vi "ConvertGoop3ToGoop4_SelectNodesToBeInsideIP.vi"(1 "NodesIn":cluster{"NodesIn":T3[]}[](array[cluster]), 5 "BundleNodes":cluster{"BundleNodes":refnum<vi>[]}[](array[cluster]), 9 "BundleNodeTypes":cluster{"BundleNodeTypes":string[]}[](array[cluster]), 11 "error in":errorcluster, 12 "GetAttribute_AttributeTerminal":refnum<vi>[](array[refnum]), 13 "FirstGetAttributesDrainsTerminals":refnum<vi>[](array[refnum]), 14 "LastGetAttributesSourceTerminals":refnum<vi>[](array[refnum])) -> (4 "NodesOut":cluster{"NodesIn":T3[]}[](array[cluster]), 6 "IPE-Position":T1, 8 "IPE-Frame Size":T2, 15 "error out":errorcluster)   [LabVIEW 2014]
uses:
  <resource>/Framework/Providers/Open_GDS/ClassProviders/Common/ScriptingFunctions/Scripting_NodeInfo.ctl
  <vilib>/Utility/miscctls.llb/LVBoundsTypeDef.ctl
  <vilib>/Utility/miscctls.llb/LVPositionTypeDef.ctl
panel:
  in  "SetAttributesDrainsTerminals":refnum<vi>[](array[refnum])
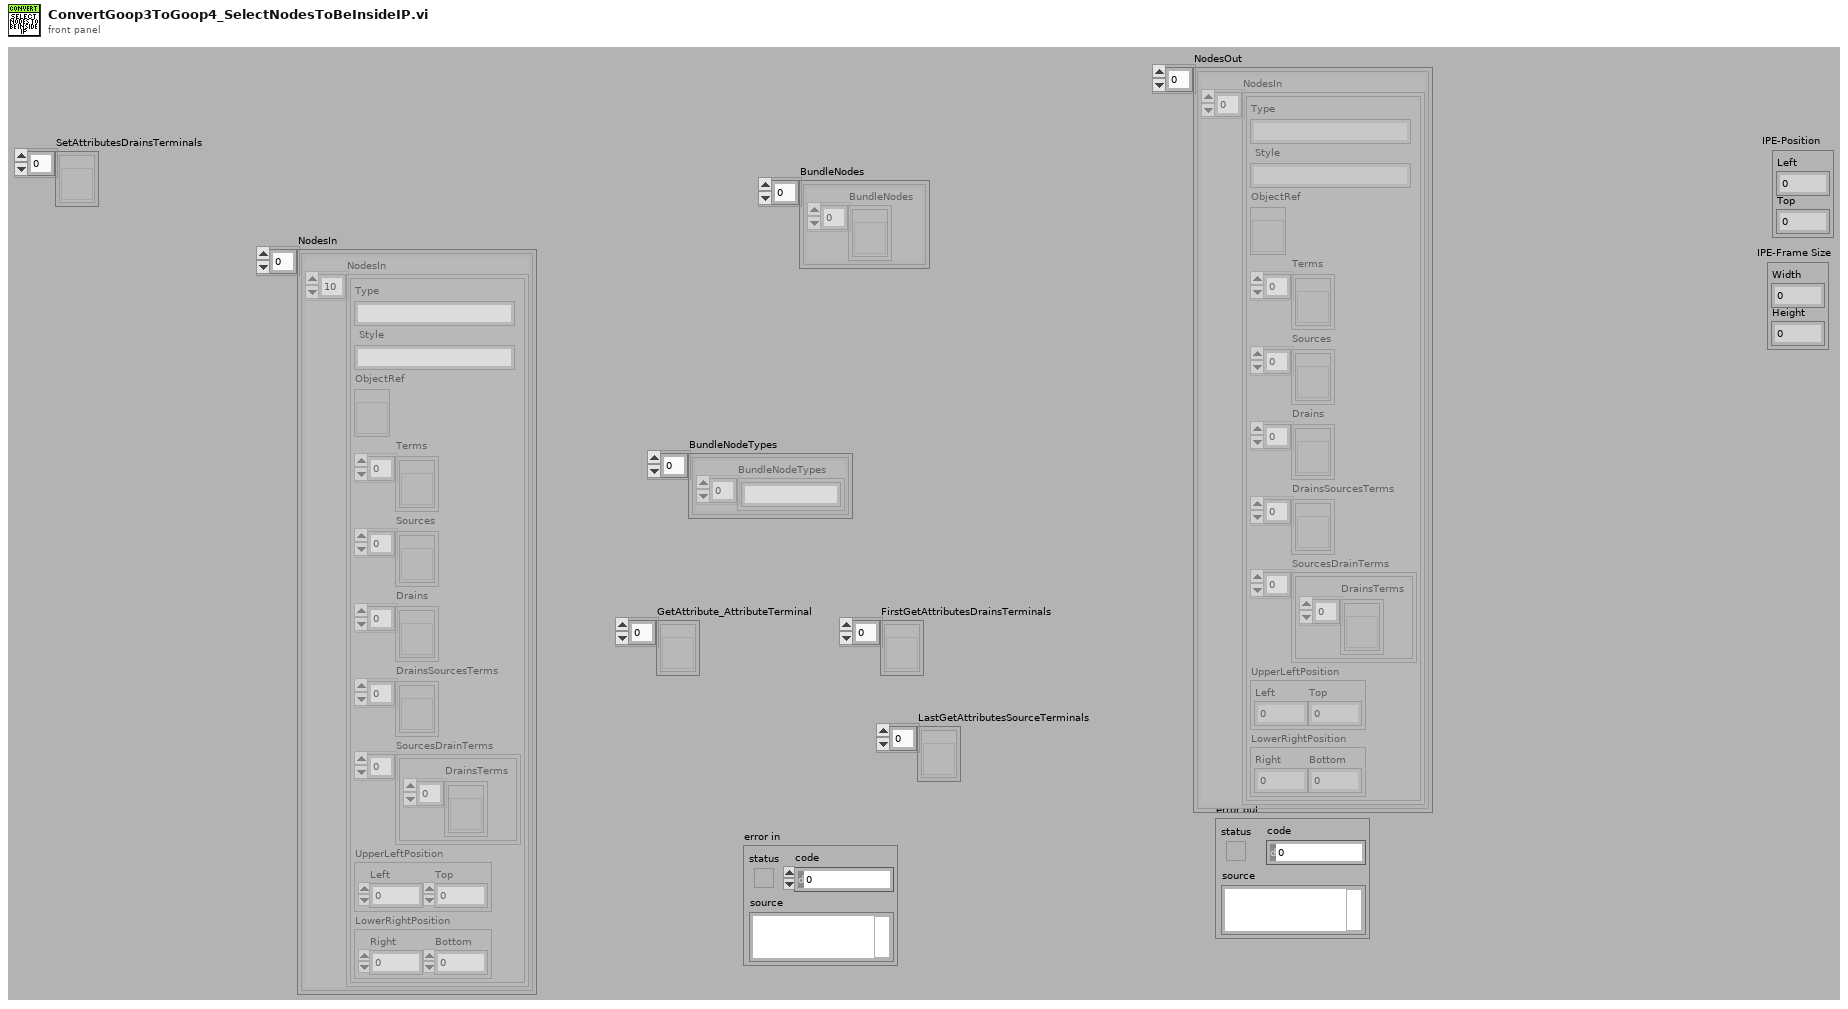
[diagram p1: front panel]
types:
  T1 = typedef "LVPositionTypeDef.ctl" = cluster{"Left":i32, "Top":i32}
  T2 = typedef "LVBoundsTypeDef.ctl" = cluster{"Width":u32, "Height":u32}
  T3 = typedef "Scripting_NodeInfo.ctl" = cluster{"Type":string, "Style":string, "ObjectRef":refnum<vi>, "Terms":refnum<vi>[], "Sources":refnum<vi>[], "Drains":refnum<vi>[], "DrainsSourcesTerms":refnum<vi>[], "SourcesDrainTerms":cluster{"DrainsTerms":refnum<vi>[]}[], "UpperLeftPosition":cluster{"Left":i32, "Top":i32}, "LowerRightPosition":cluster{"Right":i32, "Bottom":i32}}
  T4 = cluster{"SourcesDrainTerms":cluster{"DrainsTerms":refnum<vi>[]}[]}[]
  T5 = cluster{"SourcesDrainTerms":cluster{"DrainsTerms":refnum<vi>[]}[]}
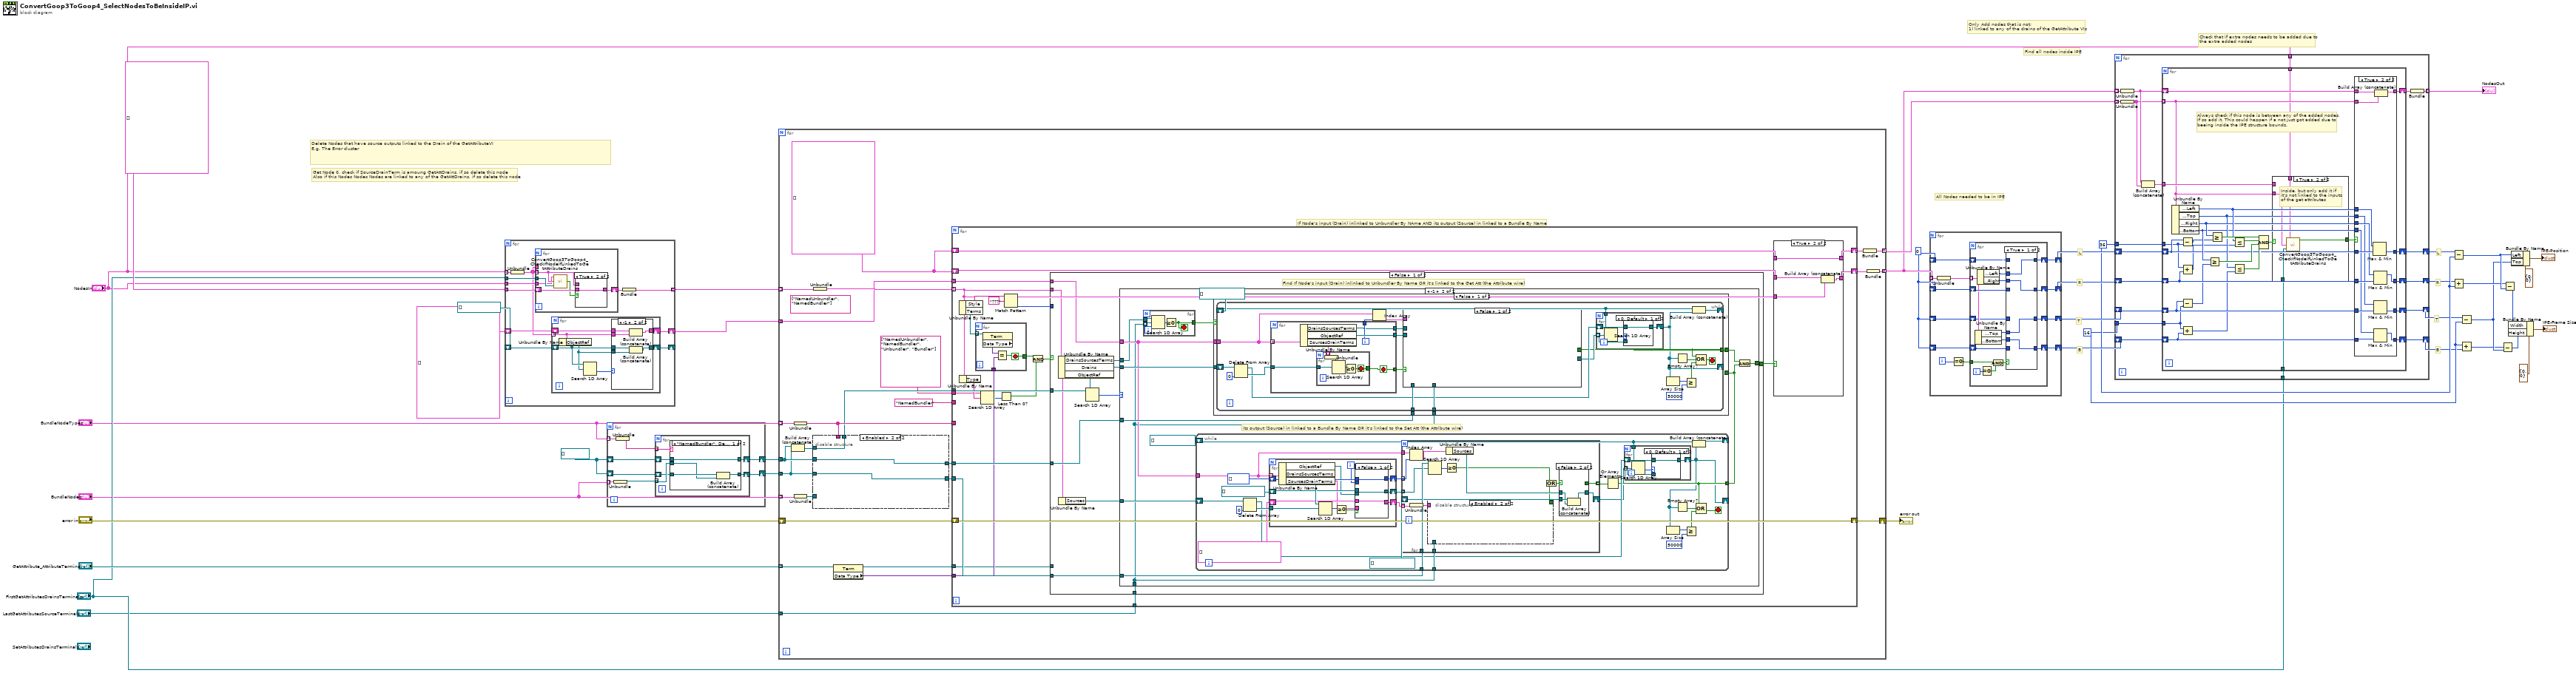
[diagram p0: block diagram]
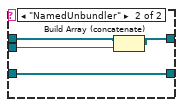
[diagram p2: hidden frame]
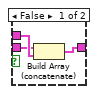
[diagram p4: hidden frame]
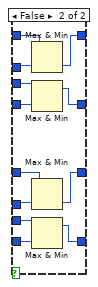
[diagram p7: hidden frame]
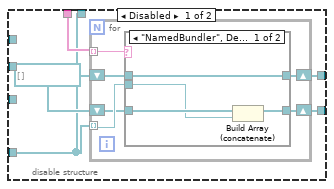
[diagram p8: hidden frame]
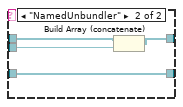
[diagram p9: hidden frame]
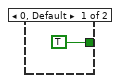
[diagram p10: hidden frame]
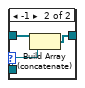
[diagram p11: hidden frame]
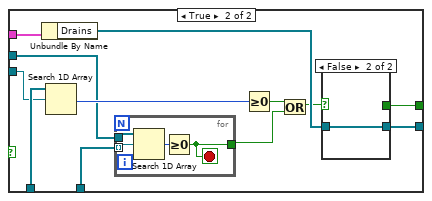
[diagram p12: hidden frame]
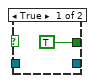
[diagram p13: hidden frame]
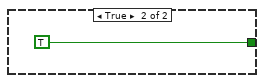
[diagram p14: hidden frame]
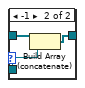
[diagram p15: hidden frame]
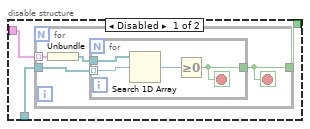
[diagram p16: hidden frame]
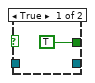
[diagram p17: hidden frame]
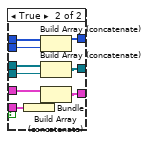
[diagram p18: hidden frame]
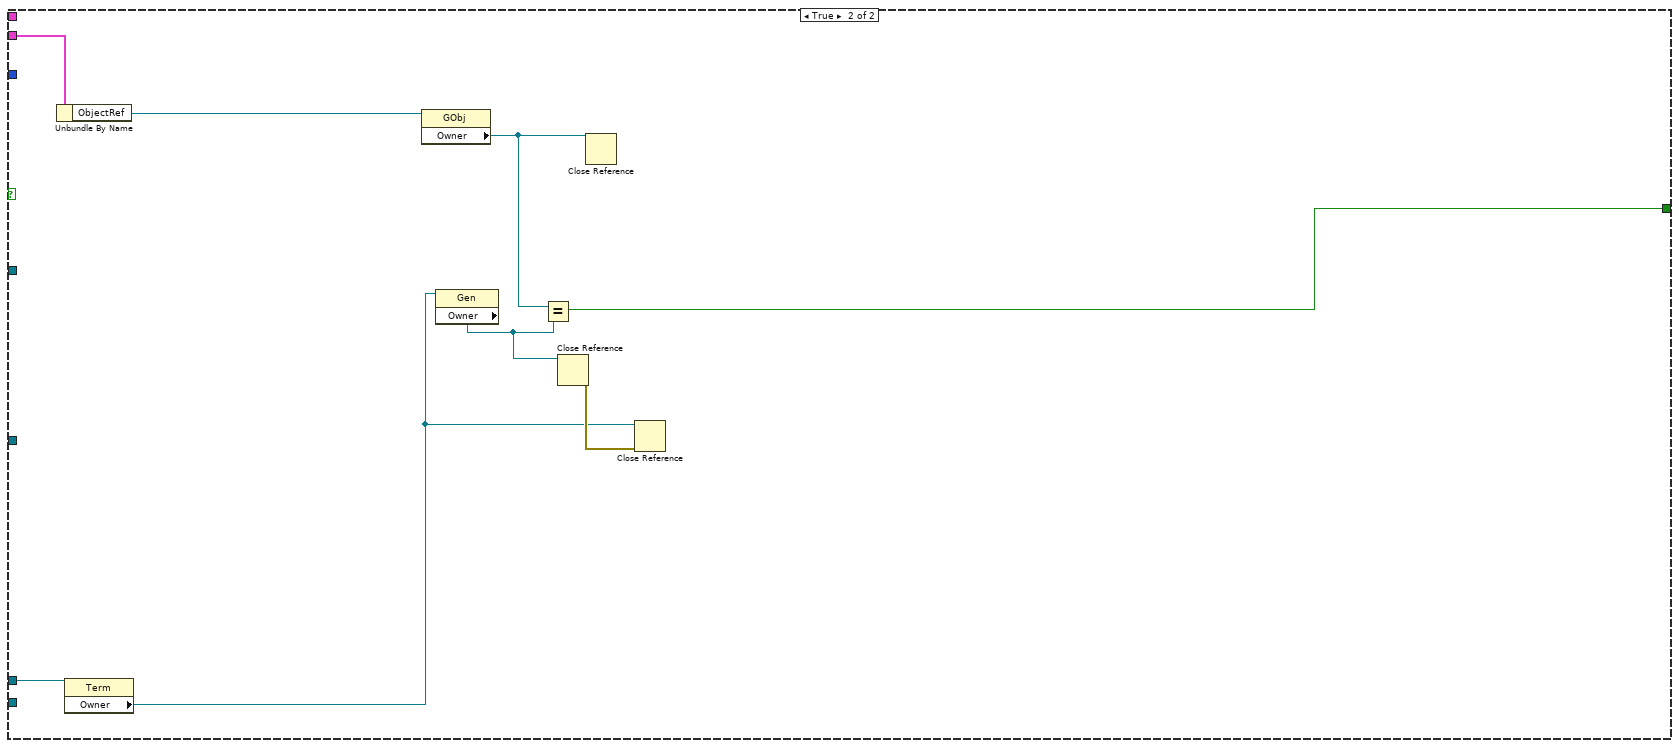
[diagram p19: hidden frame]
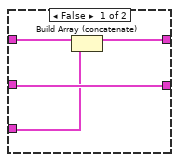
[diagram p20: hidden frame]
diagram:
  w7 = refnum<vi>[] []
  w19 = 16 ("y")
  w26 = 36 ("y")
  w15 = 0 ("Right")
  # "Get Node 0, check if SourceDrainTerm is amoung GetAttDrains, if so delete this node\nAlso if this Nodes Nodes Nodes are linked to any of the GetAttDrains, if so delete this node"
  # "Delete Nodes that have source outputs linked to the Drain of the GetAttributeVI\nE.g. The Error cluster"
  # "Check that if extra nodes needs to be added due to\nthe extra added nodes"
  # "Only Add nodes that is not:\n1) linked to any of the drains of the GetAttribute VIs"
  # "B"
  # "T"
  # "R"
  # "L"
  # "Find all nodes inside IPE"
  # "B"
  # "T"
  # "R"
  # "L"
  # "All Nodes needed to be in IPE"
  n1 = for {
    tunnel: "NodesIn" -> [w51] mode=indexing
    tunnel: [w49] -> w13 mode=indexing
    tunnel: T3[] [] -> [w48]
    tunnel: "FirstGetAttributesDrainsTerminals" -> [w47]
    tunnel: "NodesIn" -> [w46]
    shift-right: [w45] -> w2
    shift-left: T3[] [] -> [w44]
    shift-right: [w42] -> _
    shift-left: refnum<vi>[] [] -> [w43]
    n2 = Unbundle(w51) -> ("NodesIn"=w41:T3[])
    n3 = for {
      tunnel: w41 -> [w72] mode=indexing
      shift-right: [w71] -> w50
      shift-left: w48 -> [w70]
      tunnel: w41 -> [_]
      tunnel: w47 -> [w68]
      tunnel: w46 -> [w67]
      n4 = call <resource>:"ConvertGoop3ToGoop4_CheckIfNodeIfLinkedToGetAttributeDrains.vi"("FirstGetAttributesDrainsTerminals"=w68, "NodeInfo"=w72, "NodesIn"=w67) -> ("Boolean"=w69:bool)
      n5 = case shown="True" w69 {
        tunnel: w72 -> [w75 _]
        tunnel: [w74 w76] -> w71
        tunnel: w70 -> [w73 w76]
        frame False {
          n6 = Build Array (concatenate)(w73, w75) -> (w74:T3[])
        }
        frame True {
        }
      }
    }
    n7 = for {
      tunnel: w41 -> [w55] mode=indexing
      shift-right: [w58] -> w45
      shift-left: w44 -> [w57]
      shift-right: [w56] -> w42
      shift-left: w43 -> [w54]
      n8 = Unbundle By Name(w55) -> ("ObjectRef"=w53:refnum<vi>)
      n9 = Search 1D Array(1D array=w54, element=w53) -> (index of element=w52:i32)  [unwired: 1 in]
      n10 = case shown="-1" w52 {
        tunnel: [w60 w66] -> w58
        tunnel: w57 -> [w60 w65]
        tunnel: [w59 w64] -> w56
        tunnel: w55 -> [_ w63]
        tunnel: w54 -> [w59 w62]
        tunnel: w53 -> [_ w61]
        frame 0, Default {
        }
        frame -1 {
          n11 = Build Array (concatenate)(w65, w63) -> (w66:T3[])
          n12 = Build Array (concatenate)(w62, w61) -> (w64:refnum<vi>[])
        }
      }
    }
    n13 = Bundle(w50) -> (w49:cluster{T3[]})  [unwired: 1 in]
  }
  n14 = for {
    tunnel: "BundleNodes" -> [w84] mode=indexing
    shift-right: [w80] -> w5
    shift-left: w7 -> [w82]
    shift-right: [w79] -> w4
    shift-left: w7 -> [w81]
    tunnel: "BundleNodeTypes" -> [w78] mode=indexing
    n15 = Unbundle(w84) -> ("BundleNodes"=w83:refnum<vi>[])
    n16 = Unbundle(w78) -> ("BundleNodeTypes"=w77:string[])
    n17 = for {
      tunnel: w77 -> [w90] mode=indexing
      tunnel: w83 -> [w87] mode=indexing
      shift-right: [w88] -> w80
      shift-left: w82 -> [w89]
      shift-right: [w86] -> w79
      shift-left: w81 -> [w85]
      n18 = case shown="\"NamedBundler\", Default" w90 {
        tunnel: w89 -> [w94 w98]
        tunnel: [w94 w97] -> w88
        tunnel: w87 -> [w91 w96]
        tunnel: w85 -> [w93 w95]
        tunnel: [w92 w95] -> w86
        frame "NamedBundler", Default {
          n19 = Build Array (concatenate)(w93, w91) -> (w92:refnum<vi>[])
        }
        frame "NamedUnbundler" {
          n20 = Build Array (concatenate)(w98, w96) -> (w97:refnum<vi>[])
        }
      }
    }
  }
  n21 = for {
    tunnel: w13 -> [w119] mode=indexing
    tunnel: "BundleNodeTypes" -> [w117] mode=indexing
    tunnel: "BundleNodes" -> [w115] mode=indexing
    tunnel: [w110] -> w39 mode=indexing
    tunnel: [w112] -> w36 mode=indexing
    shift-right: [w124] -> w40
    shift-left: "error in" -> [w120]
    tunnel: "GetAttribute_AttributeTerminal" -> [w109] mode=indexing
    tunnel: "LastGetAttributesSourceTerminals" -> [w106]
    tunnel: w5 -> [w105]
    tunnel: w4 -> [w104]
    tunnel: w2 -> [w101]
    (unwired) string[] ["NamedUnbundler", "NamedBundler"]
    w121 = T3[] []
    # "If Node's input (Drain) inlinked to Unbundler By NAme AND its output (Source) in linked to a Bundle By Name"
    n22 = Build Array (concatenate)(w105, w104) -> (w103:refnum<vi>[])
    n23 = Unbundle(w117) -> ("BundleNodeTypes"=w116:string[])
    n24 = Unbundle(w115) -> ("BundleNodes"=w114:refnum<vi>[])
    n25 = disable-structure shown="Enabled" {
      disable-tunnel: [w128 w146] -> w123
      disable-tunnel: [w127 w145] -> w122
      disable-tunnel: w116 -> [w126 _]
      disable-tunnel: w114 -> [w125 _]
      disable-tunnel: w105 -> [_ w146]
      disable-tunnel: w104 -> [_ w145]
      disable-tunnel: w103 -> [_ w144]
      disable-tunnel: [w125 w144] -> w102
      frame Disabled {
        w129 = refnum<vi>[] []
        n26 = for {
          tunnel: w126 -> [w135] mode=indexing
          tunnel: w125 -> [w132] mode=indexing
          shift-right: [w133] -> w128
          shift-left: w129 -> [w134]
          shift-right: [w131] -> w127
          shift-left: w129 -> [w130]
          n27 = case shown="\"NamedBundler\", Default" w135 {
            tunnel: w134 -> [w139 w143]
            tunnel: [w139 w142] -> w133
            tunnel: w132 -> [w136 w141]
            tunnel: w130 -> [w138 w140]
            tunnel: [w137 w140] -> w131
            frame "NamedBundler", Default {
              n28 = Build Array (concatenate)(w138, w136) -> (w137:refnum<vi>[])
            }
            frame "NamedUnbundler" {
              n29 = Build Array (concatenate)(w143, w141) -> (w142:refnum<vi>[])
            }
          }
        }
      }
      frame Enabled {
      }
    }
    n30 = Unbundle(w119) -> (w118:T3[])
    n31 = property class="Term"(reference=w109) -> (reference out=w107:refnum<vi>, "Data Type"=w108:variant)  [unwired: 1 in, 1 out]
    n32 = for {
      tunnel: w118 -> [w153] mode=indexing
      tunnel: w116 -> [_]
      shift-right: [w170] -> w124
      shift-left: w120 -> [w170]
      shift-right: [w169] -> w113
      shift-left: w121 -> [w168]
      tunnel: w101 -> [w167]
      tunnel: w123 -> [w166]
      tunnel: w122 -> [w163]
      tunnel: w102 -> [w164]
      shift-right: [w162] -> w111
      shift-left: w121 -> [w161]
      tunnel: w108 -> [w159]
      tunnel: w107 -> [w158]
      tunnel: w106 -> [w157]
      tunnel: "NamedBundler" ("regular expression") -> [_]
      tunnel: string[] ["NamedUnbundler", "NamedBundler", "Unbundler", "Bundler"] -> [w149]
      n33 = Unbundle By Name(w153) -> ("Style"=w156:string, "Terms"=w160:refnum<vi>[])
      n34 = Unbundle By Name(w153) -> ("Type"=w150:string)
      n35 = for {
        tunnel: w160 -> [w371] mode=indexing
        tunnel: w159 -> [w369]
        tunnel: [w368] -> w152
        stop <- w368 stop-if-true
        n36 = property class="Term"(reference=w371) -> ("Data Type"=w370:variant)  [unwired: 1 in, 2 out]
        n37 = Equal?(x=w370, y=w369) -> (x = y?=w368:bool)
      }
      n38 = Search 1D Array(1D array=w149, element=w150) -> (index of element=w148:i32)  [unwired: 1 in]
      n39 = Less Than 0?(x=w148) -> (x < 0?=w147:bool)
      n40 = Match Pattern(string=w156, regular expression="???") -> (offset past match=w154:i32)  [unwired: 1 in, 3 out]
      n41 = And(x=w152, y=w147) -> (x .and. y?=w151:bool)
      n42 = case shown="False" w151 {
        tunnel: w167 -> [w181 _]
        tunnel: w166 -> [w180 _]
        tunnel: [w179 w364] -> w165
        tunnel: w164 -> [w178 _]
        tunnel: w163 -> [w174 _]
        tunnel: w153 -> [w173 w367]
        tunnel: w158 -> [_ w365]
        tunnel: w157 -> [w171 _]
        tunnel: w154 -> [_ _]
        frame False {
          # "Find If Node's input (Drain) inlinked to Unbundler By Name OR it's linked to the Get Att (the Attribute wire)"
          n43 = Unbundle By Name(w173) -> ("DrainsSourcesTerms"=w172:refnum<vi>[], "Drains"=w182:refnum<vi>[], "ObjectRef"=w177:refnum<vi>)
          n44 = Unbundle By Name(w173) -> ("Sources"=w175:refnum<vi>[])
          n45 = Search 1D Array(1D array=w178, element=w177) -> (index of element=w176:i32)  [unwired: 1 in]
          n46 = case shown="-1" w176 {
            tunnel: w182 -> [_ w195]
            tunnel: w181 -> [_ w192]
            tunnel: w180 -> [_ w193]
            tunnel: [TRUE w194] -> w179
            tunnel: w175 -> [_ w191]
            tunnel: w174 -> [_ w190]
            tunnel: w172 -> [_ w188]
            tunnel: w171 -> [_ w186]
            frame 0, Default {
            }
            frame -1 {
              # "its output (Source) in linked to a Bundle By Name OR it's linked to the Set Att (the Attribute wire)"
              n47 = for {
                tunnel: w188 -> [w267]
                tunnel: w186 -> [w266] mode=indexing
                tunnel: [w264] -> w187
                stop <- w264 stop-if-true
                n48 = Search 1D Array(1D array=w267, element=w266) -> (index of element=w265:i32)  [unwired: 1 in]
                n49 = Greater Or Equal To 0?(x=w265) -> (x >= 0?=w264:bool)
              }
              n50 = while {
                tunnel: w192 -> [w287]
                tunnel: w190 -> [w292]
                tunnel: [w270] -> w185
                shift-right: [w269] -> _
                shift-left: w191 -> [w291]
                tunnel: w186 -> [w279]
                shift-right: [w278] -> _
                shift-left: refnum<vi>[] [] -> [w277]
                stop <- w271 stop-if-true
                n51 = Delete From Array(array=w291, index=0) -> (deleted portion=w288:refnum<vi>, array with subset deleted=w276:refnum<vi>[])  [unwired: 1 in]
                n52 = for {
                  tunnel: w287 -> [w346] mode=indexing
                  tunnel: w288 -> [w345]
                  shift-right: [w341] -> w286
                  shift-left: i32[] [] -> [w340]
                  shift-right: [w338] -> w285
                  shift-left: refnum<vi>[] [] -> [w339]
                  shift-right: [w333] -> w280
                  shift-left: T4 [] -> [w335]
                  i -> [w337]
                  n53 = Unbundle By Name(w346) -> ("ObjectRef"=w336:refnum<vi>, "DrainsSourcesTerms"=w343:refnum<vi>[], "SourcesDrainTerms"=w334:cluster{"DrainsTerms":refnum<vi>[]}[])
                  n54 = Search 1D Array(1D array=w343, element=w345) -> (index of element=w344:i32)  [unwired: 1 in]
                  n55 = Greater Or Equal To 0?(x=w344) -> (x >= 0?=w342:bool)
                  n56 = case shown="False" w342 {
                    tunnel: [w349 w359] -> w341
                    tunnel: w340 -> [w349 w358]
                    tunnel: w339 -> [w348 w357]
                    tunnel: [w348 w356] -> w338
                    tunnel: w337 -> [_ w355]
                    tunnel: w336 -> [_ w354]
                    tunnel: w335 -> [w347 w352]
                    tunnel: [w347 w353] -> w333
                    tunnel: w334 -> [_ w351]
                    frame False {
                    }
                    frame True {
                      n57 = Bundle("SourcesDrainTerms"=w351) -> (w350:T5)  [unwired: 1 in]
                      n58 = Build Array (concatenate)(w358, w355) -> (w359:i32[])
                      n59 = Build Array (concatenate)(w357, w354) -> (w356:refnum<vi>[])
                      n60 = Build Array (concatenate)(w352, w350) -> (w353:T4)
                    }
                  }
                }
                n61 = for {
                  tunnel: w292 -> [w317]
                  tunnel: [w316] -> w289 mode=indexing
                  tunnel: w287 -> [w313]
                  tunnel: w286 -> [w312] mode=indexing
                  tunnel: w285 -> [w310] mode=indexing
                  shift-right: [w315] -> w268
                  shift-left: refnum<vi>[] [] -> [w309]
                  tunnel: w280 -> [w305] mode=indexing
                  tunnel: w279 -> [w303]
                  n62 = Unbundle(w305) -> ("SourcesDrainTerms"=w304:cluster{"DrainsTerms":refnum<vi>[]}[])
                  n63 = Index Array(array=w313, index=w312) -> (element=w311:T3)
                  n64 = disable-structure shown="Enabled" {
                    disable-tunnel: w304 -> [w320 _]
                    disable-tunnel: w303 -> [w319 _]
                    disable-tunnel: [w318 _] -> w302
                    frame Disabled {
                      n65 = for {
                        tunnel: w320 -> [w324] mode=indexing
                        tunnel: w319 -> [w322]
                        tunnel: [w321] -> w318
                        stop <- w321 stop-if-true
                        n66 = Unbundle(w324) -> ("DrainsTerms"=w323:refnum<vi>[])
                        n67 = for {
                          tunnel: w323 -> [w328]
                          tunnel: w322 -> [w327] mode=indexing
                          tunnel: [w325] -> w321
                          stop <- w325 stop-if-true
                          n68 = Search 1D Array(1D array=w328, element=w327) -> (index of element=w326:i32)  [unwired: 1 in]
                          n69 = Greater Or Equal To 0?(x=w326) -> (x >= 0?=w325:bool)
                        }
                      }
                    }
                    frame Enabled {
                    }
                  }
                  n70 = Search 1D Array(1D array=w317, element=w310) -> (index of element=w308:i32)  [unwired: 1 in]
                  n71 = Greater Or Equal To 0?(x=w308) -> (x >= 0?=w307:bool)
                  n72 = Unbundle By Name(w311) -> ("Sources"=w314:refnum<vi>[])
                  n73 = Or(x=w307, y=w302) -> (x .or. y?=w306:bool)
                  n74 = case shown="False" w306 {
                    tunnel: [TRUE _] -> w316
                    tunnel: [_ w330] -> w315
                    tunnel: w314 -> [_ w331]
                    tunnel: w309 -> [_ w332]
                    frame True {
                    }
                    frame False {
                      n75 = Build Array (concatenate)(w332, w331) -> (w330:refnum<vi>[])
                    }
                  }
                }
                n76 = Or Array Elements(Boolean array=w289) -> (logical OR=w270:bool)
                n77 = for {
                  shift-right: [w296] -> w269
                  shift-left: w276 -> [w297]
                  tunnel: w268 -> [w295] mode=indexing
                  tunnel: w277 -> [w293]
                  n78 = Search 1D Array(1D array=w293, element=w295) -> (index of element=w294:i32)  [unwired: 1 in]
                  n79 = case shown="0, Default" w294 {
                    tunnel: w297 -> [w298 w301]
                    tunnel: [w298 w300] -> w296
                    tunnel: w295 -> [_ w299]
                    frame 0, Default {
                    }
                    frame -1 {
                      n80 = Build Array (concatenate)(w301, w299) -> (w300:refnum<vi>[])
                    }
                  }
                }
                n81 = Array Size(array=w269) -> (size(s)=w272:i32)
                n82 = Empty Array?(array=w269) -> (empty?=w275:bool)
                n83 = Greater Or Equal?(x=w272, y=50000) -> (x >= y?=w274:bool)
                n84 = Build Array (concatenate)(w277, w269) -> (w278:refnum<vi>[])
                n85 = Compound Arithmetic op=OR(w270, w275, w274) -> (w271:bool)
              }
              n86 = case shown="False" w187 {
                tunnel: w195 -> [w201 _]
                tunnel: w193 -> [w200 _]
                tunnel: w192 -> [w199 _]
                tunnel: [w198 TRUE] -> w189
                tunnel: w186 -> [w197 _]
                tunnel: w185 -> [_ _]
                frame False {
                  n87 = while {
                    tunnel: w199 -> [w217]
                    tunnel: w200 -> [w221]
                    tunnel: [w204] -> w198
                    shift-right: [w202] -> _
                    shift-left: w201 -> [w220]
                    tunnel: w197 -> [w214]
                    shift-right: [w212] -> _
                    shift-left: refnum<vi>[] [] -> [w211]
                    stop <- w203 stop-if-true
                    n88 = Delete From Array(array=w220, index=0) -> (deleted portion=w215:refnum<vi>, array with subset deleted=w210:refnum<vi>[])  [unwired: 1 in]
                    n89 = for {
                      tunnel: w217 -> [w257] mode=indexing
                      tunnel: w215 -> [w255]
                      tunnel: [w252] -> w223
                      tunnel: [w254] -> w222
                      tunnel: [w253] -> w218
                      tunnel: [w251] -> w213
                      i -> [w253]
                      stop <- w252 stop-if-true
                      n90 = Unbundle By Name(w257) -> ("DrainsSourcesTerms"=w251:refnum<vi>[], "ObjectRef"=w254:refnum<vi>, "SourcesDrainTerms"=w256:cluster{"DrainsTerms":refnum<vi>[]}[])
                      n91 = for {
                        tunnel: w256 -> [w261] mode=indexing
                        tunnel: w255 -> [w262]
                        tunnel: [w258] -> w252
                        stop <- w258 stop-if-true
                        n92 = Unbundle(w261) -> ("DrainsTerms"=w260:refnum<vi>[])
                        n93 = Search 1D Array(1D array=w260, element=w262) -> (index of element=w259:i32)  [unwired: 1 in]
                        n94 = Greater Or Equal To 0?(x=w259) -> (x >= 0?=w258:bool)
                      }
                    }
                    n95 = Index Array(array=w217, index=w218) -> (element=w216:T3)
                    n96 = case shown="False" w223 {
                      tunnel: w222 -> [_ w243]
                      tunnel: w221 -> [_ w244]
                      tunnel: [_ w242] -> w204
                      tunnel: [_ w241] -> w209
                      tunnel: w216 -> [_ w240]
                      tunnel: w214 -> [_ w233]
                      tunnel: w213 -> [_ w234]
                      frame False {
                      }
                      frame True {
                        n97 = Unbundle By Name(w240) -> ("Drains"=w239:refnum<vi>[])
                        n98 = Search 1D Array(1D array=w244, element=w243) -> (index of element=w238:i32)  [unwired: 1 in]
                        n99 = for {
                          tunnel: w234 -> [w248]
                          tunnel: w233 -> [w247] mode=indexing
                          tunnel: [w245] -> w235
                          stop <- w245 stop-if-true
                          n100 = Search 1D Array(1D array=w248, element=w247) -> (index of element=w246:i32)  [unwired: 1 in]
                          n101 = Greater Or Equal To 0?(x=w246) -> (x >= 0?=w245:bool)
                        }
                        n102 = Greater Or Equal To 0?(x=w238) -> (x >= 0?=w237:bool)
                        n103 = Or(x=w237, y=w235) -> (x .or. y?=w236:bool)
                        n104 = case shown="False" w236 {
                          tunnel: [TRUE _] -> w242
                          tunnel: [_ w250] -> w241
                          tunnel: w239 -> [_ w250]
                          frame True {
                          }
                          frame False {
                          }
                        }
                      }
                    }
                    n105 = for {
                      shift-right: [w227] -> w202
                      shift-left: w210 -> [w228]
                      tunnel: w209 -> [w226] mode=indexing
                      tunnel: w211 -> [w224]
                      n106 = Search 1D Array(1D array=w224, element=w226) -> (index of element=w225:i32)  [unwired: 1 in]
                      n107 = case shown="0, Default" w225 {
                        tunnel: w228 -> [w229 w232]
                        tunnel: [w229 w231] -> w227
                        tunnel: w226 -> [_ w230]
                        frame 0, Default {
                        }
                        frame -1 {
                          n108 = Build Array (concatenate)(w232, w230) -> (w231:refnum<vi>[])
                        }
                      }
                    }
                    n109 = Array Size(array=w202) -> (size(s)=w208:i32)
                    n110 = Empty Array?(array=w202) -> (empty?=w205:bool)
                    n111 = Greater Or Equal?(x=w208, y=50000) -> (x >= y?=w206:bool)
                    n112 = Build Array (concatenate)(w211, w202) -> (w212:refnum<vi>[])
                    n113 = Compound Arithmetic op=OR(w204, w205, w206) -> (w203:bool)
                  }
                }
                frame True {
                }
              }
              n114 = And(x=w189, y=w185) -> (x .and. y?=w194:bool)
            }
          }
        }
        frame True {
          n115 = Unbundle By Name(w367) -> ("ObjectRef"=w366:refnum<vi>)
          n116 = property class="Term"(reference=w365) -> ("Owner"=w360:refnum<vi>)  [unwired: 1 in, 2 out]
          n117 = property class="GObj"(reference=w366) -> ("Owner"=w363:refnum<vi>)  [unwired: 1 in, 2 out]
          n118 = property class="Gen"(reference=w360) -> ("Owner"=w362:refnum<vi>)  [unwired: 1 in, 2 out]
          n119 = Equal?(x=w363, y=w362) -> (x = y?=w364:bool)
          n120 = Close Reference(reference=w362) -> (error out=w361:errorcluster)  [unwired: 1 in]
          n121 = Close Reference(reference=w363) -> ()  [unwired: 1 in, 1 out]
          n122 = Close Reference(reference=w360, error in (no error)=w361) -> ()  [unwired: 1 out]
        }
      }
      n123 = case shown="True" w165 {
        tunnel: [w375 w379] -> w169
        tunnel: w168 -> [w375 w378]
        tunnel: w153 -> [w372 w377]
        tunnel: [w374 w376] -> w162
        tunnel: w161 -> [w373 w376]
        frame False {
          n124 = Build Array (concatenate)(w373, w372) -> (w374:T3[])
        }
        frame True {
          n125 = Build Array (concatenate)(w378, w377) -> (w379:T3[])
        }
      }
    }
    n126 = Bundle(w111) -> (w110:cluster{T3[]})  [unwired: 1 in]
    n127 = Bundle(w113) -> (w112:cluster{T3[]})  [unwired: 1 in]
  }
  "error out" <- w40
  n128 = for {
    tunnel: w36 -> [w386] mode=indexing
    shift-right: [w388] -> w34
    shift-left: w15 -> [w382]
    shift-right: [w387] -> w33
    shift-left: w15 -> [w383]
    shift-right: [w390] -> w38
    shift-left: w15 -> [w384]
    shift-right: [w389] -> w37
    shift-left: w15 -> [w391]
    i -> [w381]
    n129 = Unbundle(w386) -> (w385:T3[])
    n130 = Equal To 0?(x=w381) -> (x = 0?=w380:bool)
    n131 = for {
      tunnel: w385 -> [w402] mode=indexing
      shift-right: [w406] -> w387
      shift-left: w383 -> [w407]
      shift-right: [w405] -> w388
      shift-left: w382 -> [w403]
      shift-right: [w399] -> w389
      shift-left: w391 -> [w396]
      shift-right: [w400] -> w390
      shift-left: w384 -> [w401]
      tunnel: w380 -> [w394]
      i -> [w395]
      n132 = Unbundle By Name(w402) -> ("UpperLeftPosition.Top"=w398:i32, "LowerRightPosition.Bottom"=w397:i32)
      n133 = Unbundle By Name(w402) -> ("UpperLeftPosition.Left"=w404:i32, "LowerRightPosition.Right"=w408:i32)
      n134 = Equal To 0?(x=w395) -> (x = 0?=w393:bool)
      n135 = And(x=w394, y=w393) -> (x .and. y?=w392:bool)
      n136 = case shown="True" w392 {
        tunnel: w408 -> [w412 w424]
        tunnel: w407 -> [_ w423]
        tunnel: [w412 w422] -> w406
        tunnel: [w411 w420] -> w405
        tunnel: w404 -> [w411 w421]
        tunnel: w403 -> [_ w419]
        tunnel: w397 -> [w409 w413]
        tunnel: w396 -> [_ w414]
        tunnel: [w409 w415] -> w399
        tunnel: [w410 w417] -> w400
        tunnel: w398 -> [w410 w416]
        tunnel: w401 -> [_ w418]
        frame True {
        }
        frame False {
          n137 = Max & Min(x=w419, y=w421) -> (min(x,y)=w420:i32)  [unwired: 1 out]
          n138 = Max & Min(x=w424, y=w423) -> (max(x,y)=w422:i32)  [unwired: 1 out]
          n139 = Max & Min(x=w418, y=w416) -> (min(x,y)=w417:i32)  [unwired: 1 out]
          n140 = Max & Min(x=w413, y=w414) -> (max(x,y)=w415:i32)  [unwired: 1 out]
        }
      }
    }
  }
  n141 = for {
    tunnel: w39 -> [w433] mode=indexing
    tunnel: w36 -> [w432] mode=indexing
    tunnel: [w430] -> w35 mode=indexing
    tunnel: w26 -> [w439]
    tunnel: w19 -> [w435]
    shift-right: [w434] -> w18
    shift-left: w37 -> [w442]
    shift-right: [w436] -> w21
    shift-left: w38 -> [w443]
    shift-right: [w437] -> w23
    shift-left: w33 -> [w440]
    shift-right: [w438] -> w25
    shift-left: w34 -> [w441]
    tunnel: "FirstGetAttributesDrainsTerminals" -> [w426]
    tunnel: "NodesIn" -> [w425]
    n142 = Unbundle(w432) -> (w429:T3[])
    n143 = Unbundle(w433) -> (w428:T3[])
    n144 = Build Array (concatenate)(w429, w428) -> (w427:T3[])
    n145 = for {
      tunnel: w428 -> [w447] mode=indexing
      shift-right: [w468] -> w431
      shift-left: w429 -> [w469]
      shift-right: [w464] -> w438
      shift-left: w441 -> [w459]
      shift-right: [w465] -> w437
      shift-left: w440 -> [w457]
      shift-right: [w466] -> w436
      shift-left: w443 -> [w454]
      shift-right: [w467] -> w434
      shift-left: w442 -> [w452]
      tunnel: w439 -> [w458]
      tunnel: w435 -> [w450]
      tunnel: w427 -> [w448]
      tunnel: w426 -> [w446]
      tunnel: w425 -> [w444]
      # "Always check if this node is between any of the added nodes,\nIf so add it. This could happen if a not just got added due to \nbeeing inside the IPE structure bounds."
      n146 = Unbundle By Name(w447) -> ("UpperLeftPosition.Left"=w463:i32, "UpperLeftPosition.Top"=w461:i32, "LowerRightPosition.Right"=w462:i32, "LowerRightPosition.Bottom"=w460:i32)
      n147 = Subtract(x=w459, y=w458) -> (x-y=w455:i32)
      n148 = Add(x=w458, y=w457) -> (x+y=w456:i32)
      n149 = Subtract(x=w454, y=w450) -> (x-y=w453:i32)
      n150 = Add(x=w450, y=w452) -> (x+y=w451:i32)
      n151 = Greater Or Equal?(x=w460, y=w453) -> (x >= y?=w471:bool)
      n152 = Greater Or Equal?(x=w462, y=w455) -> (x >= y?=w473:bool)
      n153 = Less Or Equal?(x=w463, y=w456) -> (x <= y?=w472:bool)
      n154 = Less Or Equal?(x=w461, y=w451) -> (x <= y?=w470:bool)
      n155 = Compound Arithmetic op=AND(w473, w472, w471, w470) -> (w449:bool)
      n156 = case shown="True" w449 {
        tunnel: w448 -> [_ _]
        tunnel: w447 -> [_ w477]
        tunnel: w446 -> [_ w476]
        tunnel: [_ w475] -> w445
        tunnel: w444 -> [_ w474]
        frame False {
        }
        frame True {
          # "Inside, but only add it if\nit's not linked to the inputs\nof the get attributes"
          n157 = call <resource>:"ConvertGoop3ToGoop4_CheckIfNodeIfLinkedToGetAttributeDrains.vi"("FirstGetAttributesDrainsTerminals"=w476, "NodeInfo"=w477, "NodesIn"=w474) -> ("Boolean"=w475:bool)
        }
      }
      n158 = case shown="True" w445 {
        tunnel: [w482 w497] -> w468
        tunnel: w469 -> [w482 w496]
        tunnel: w447 -> [_ w495]
        tunnel: w459 -> [w478 w493]
        tunnel: w457 -> [w479 w490]
        tunnel: w454 -> [w480 w487]
        tunnel: w452 -> [w481 w484]
        tunnel: [w481 w485] -> w467
        tunnel: [w480 w488] -> w466
        tunnel: [w479 w489] -> w465
        tunnel: [w478 w494] -> w464
        tunnel: w463 -> [_ w492]
        tunnel: w462 -> [_ w491]
        tunnel: w461 -> [_ w486]
        tunnel: w460 -> [_ w483]
        frame False {
        }
        frame True {
          n159 = Max & Min(x=w492, y=w493) -> (min(x,y)=w494:i32)  [unwired: 1 out]
          n160 = Max & Min(x=w491, y=w490) -> (max(x,y)=w489:i32)  [unwired: 1 out]
          n161 = Max & Min(x=w486, y=w487) -> (min(x,y)=w488:i32)  [unwired: 1 out]
          n162 = Max & Min(x=w483, y=w484) -> (max(x,y)=w485:i32)  [unwired: 1 out]
          n163 = Build Array (concatenate)(w496, w495) -> (w497:T3[])
        }
      }
    }
    n164 = Bundle(w431) -> (w430:cluster{T3[]})  [unwired: 1 in]
  }
  "NodesOut" <- w35
  n165 = Subtract(x=w25, y=w26) -> (x-y=w24:i32)
  n166 = Add(x=w23, y=w26) -> (x+y=w22:i32)
  n167 = Subtract(x=w21, y=w19) -> (x-y=w20:i32)
  n168 = Add(x=w19, y=w18) -> (x+y=w17:i32)
  n169 = Subtract(x=w17, y=w20) -> (x-y=w27:i32)
  n170 = Subtract(x=w22, y=w24) -> (x-y=w28:i32)
  n171 = Bundle By Name(cluster=T2 {"Width"=0, "Height"=0} ("IPE-Frame Size"), "Width"=w28, "Height"=w27) -> (→"IPE-Frame Size":T2)
  n172 = Bundle By Name(cluster=T1 {"Left"=0, "Top"=0} ("IPE-Position"), "Left"=w24, "Top"=w20) -> (→"IPE-Position":T1)
